vi "DataArray_Formatter.vi"(0 "PartitionArray":string[](array[string]), 1 "Temps":dbl[][](graph), 2 "FrozenFraction":dbl[](array[numeric]), 3 "FreezeTemps":dbl[](array[numeric]), 4 "Offsets":dbl[](array[numeric]), 5 "Offset Applied?":bool, 6 "input cluster":T1={"Core"={"Current VI Reference"=refnum, "Close Panel on Exit?"=FALSE}, "Image Out"=refnum, "State"=0, "Points"={"Top Left"={"X"=0.0, "Y"=0.0}, "Top Right"={"X"=0.0, "Y"=0.0}, "Bottom Left"={"X"=0.0, "Y"=0.0}, "Bottom Right"={"X"=0.0, "Y"=0.0}, "x space 2"=0.0, "y space 2"=0.0, "x_space"=0.0, "y_space"=0.0, "Pixels"=[], "Fixpoint"={"X"=0.0, "Y"=0.0}}, "img_array"=[], "Temps"=[], "Temps_Array"=[], "Scan Area"=0.0, "Fixpoint Area"=0.0, "Config"={"Freezing"={"Cutoff"=2.0, "EndIndex"=2}}, "PCR Size"=0, "ImageCount"=0, "ShowGradient"=FALSE} {"Points"."Bottom Right"."Y" format="%.2f"; "Points"."Bottom Right"."X" format="%.2f"; "Points"."Top Left"."Y" format="%.2f"; "Points"."Top Left"."X" format="%.2f"; "Points"."Top Right"."Y" format="%.2f"; "Points"."Top Right"."X" format="%.2f"; "Points"."Bottom Left"."Y" format="%.2f"; "Points"."Bottom Left"."X" format="%.2f"; "Points"."Fixpoint"."Y" format="%.2f"; "Points"."Fixpoint"."X" format="%.2f"}, 9 "MeltTemps":dbl[](array[numeric])) -> (14 "Data Array":string[][](array[string]))   [LabVIEW 2022 SP3]
uses:
  DataCluster_TCAL.ctl
  <vilib>/vision/Image Controls.llb/IMAQ Image.ctl
  TCE_Config.ctl
panel:
  out "appended array":string[][](array[string])
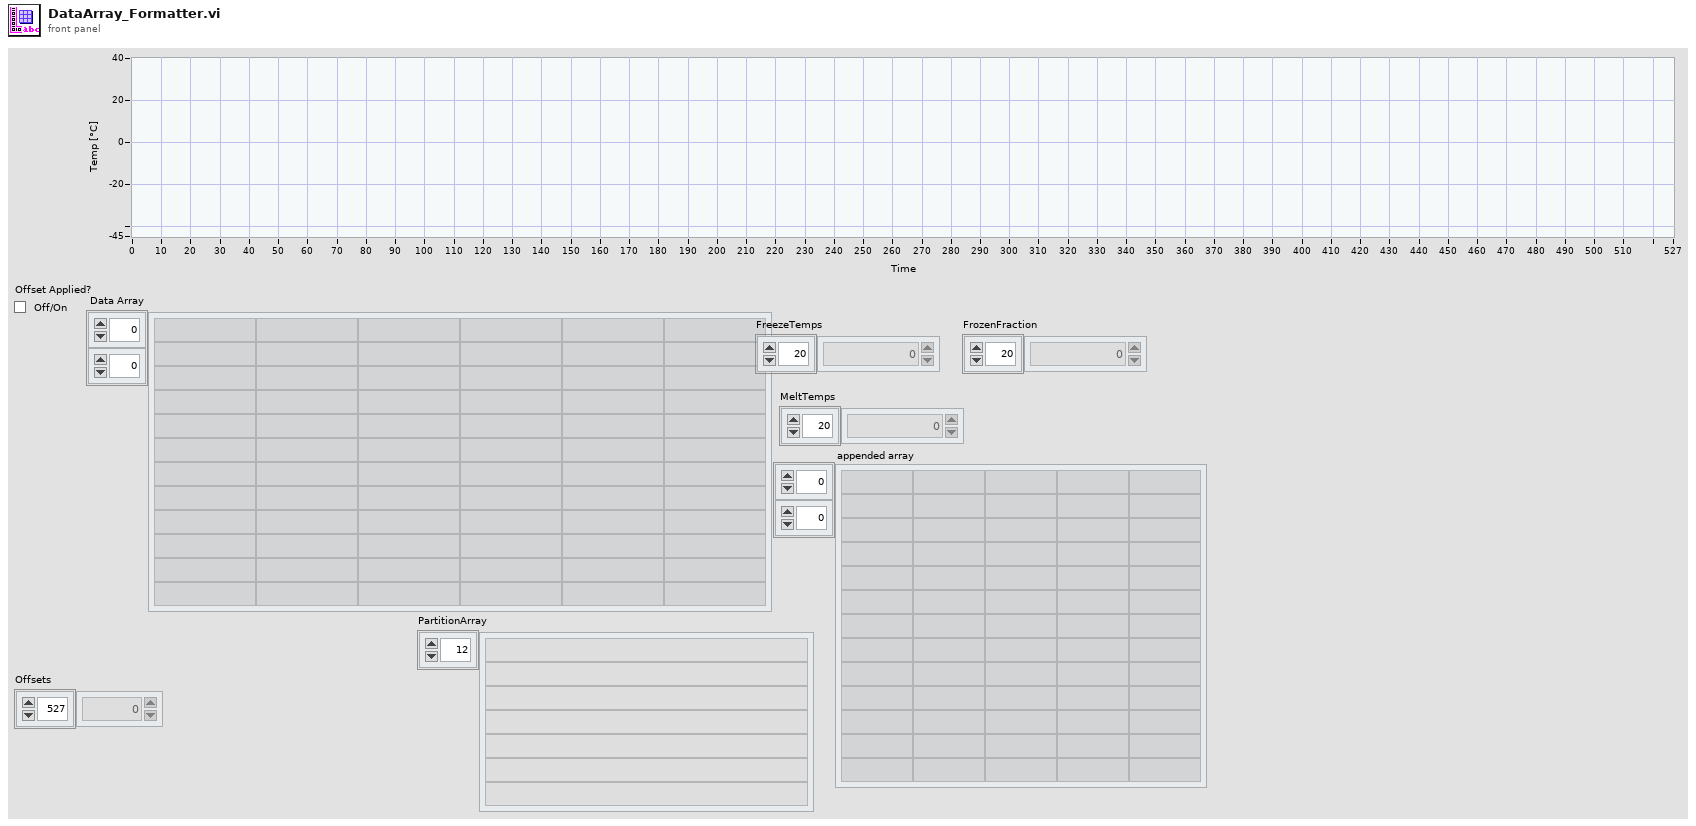
[diagram p1: front panel]
types:
  T1 = typedef "DataCluster_TCAL.ctl" = cluster{"Core":cluster{"Current VI Reference":refnum<vi>, "Close Panel on Exit?":bool}, "Image Out":T2, "State":i32, "Points":cluster{"Top Left":T3, "Top Right":T3, "Bottom Left":T3, "Bottom Right":T3, "x space 2":dbl, "y space 2":sgl, "x_space":sgl, "y_space":sgl, "Pixels":cluster{"X":i32, "Y":i32}[][], "Fixpoint":T3}, "img_array":T2[], "Temps":dbl[], "Temps_Array":dbl[][], "Scan Area":dbl, "Fixpoint Area":dbl, "Config":T4, "PCR Size":u16, "ImageCount":i32, "ShowGradient":bool}
  T2 = typedef "IMAQ Image.ctl" = refnum<image>
  T3 = typedef "IMAQ Point" = cluster{"X":sgl, "Y":sgl}
  T4 = typedef "TCE_Config.ctl" = cluster{"Freezing":cluster{"Cutoff":dbl, "EndIndex":i32}}
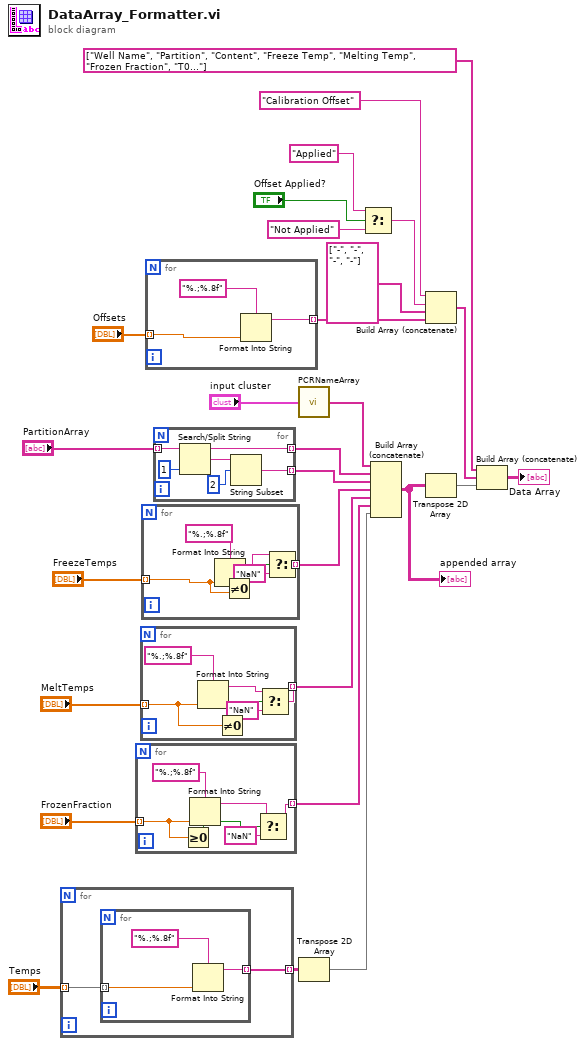
[diagram p0: block diagram]
diagram:
  n1 = for {
    tunnel: "Temps" -> [w29] mode=indexing
    tunnel: [w28] -> w21 mode=indexing
    n2 = for {
      tunnel: w29 -> [w32] mode=indexing
      tunnel: [w31] -> w28 mode=indexing
      n3 = Format Into String(format string="%.;%.8f", w32) -> (resulting string=w31:string)  [unwired: 2 in, 1 out]
    }
  }
  n4 = for {
    tunnel: "FrozenFraction" -> [w35] mode=indexing
    tunnel: [w36] -> w5 mode=indexing
    n5 = Greater Or Equal To 0?(x=w35) -> (x >= 0?=w34:bool)
    n6 = Format Into String(format string="%.;%.8f", w35) -> (resulting string=w37:string)  [unwired: 2 in, 1 out]
    n7 = Select(t=w37, s=w34, f="NaN") -> (s? t:f=w36:string)
  }
  n8 = for {
    tunnel: "MeltTemps" -> [w39] mode=indexing
    tunnel: [w42] -> w10 mode=indexing
    n9 = Format Into String(format string="%.;%.8f", w39) -> (resulting string=w41:string)  [unwired: 2 in, 1 out]
    n10 = Not Equal To 0?(x=w39) -> (x != 0?=w40:bool)
    n11 = Select(t=w41, s=w40, f="NaN") -> (s? t:f=w42:string)
  }
  n12 = for {
    tunnel: "FreezeTemps" -> [w46] mode=indexing
    tunnel: [w49] -> w3 mode=indexing
    n13 = Format Into String(format string="%.;%.8f", w46) -> (resulting string=w48:string)  [unwired: 2 in, 1 out]
    n14 = Not Equal To 0?(x=w46) -> (x != 0?=w47:bool)
    n15 = Select(t=w48, s=w47, f="NaN") -> (s? t:f=w49:string)
  }
  n16 = for {
    tunnel: "Offsets" -> [w53] mode=indexing
    tunnel: [w52] -> w9 mode=indexing
    n17 = Format Into String(format string="%.;%.8f", w53) -> (resulting string=w52:string)  [unwired: 2 in, 1 out]
  }
  n18 = for {
    tunnel: "PartitionArray" -> [w59] mode=indexing
    tunnel: [w55] -> w2 mode=indexing
    tunnel: [w57] -> w1 mode=indexing
    n19 = Search/Split String(string=w59, offset (0)=1) -> (substring before match=w57:string, match + rest of string=w56:string)  [unwired: 1 in, 1 out]
    n20 = String Subset(string=w56, offset (0)=2) -> (substring=w55:string)  [unwired: 1 in]
  }
  n21 = call "PCRNameArray.vi"("input cluster"="input cluster") -> ("WellArray"=w27:string[])
  n22 = Transpose 2D Array(2D array=w21) -> (transposed array=w6:string[][])
  n23 = Select(t="Applied", s="Offset Applied?", f="Not Applied") -> (s? t:f=w12:string)
  n24 = Build Array (concatenate)(w27, w1, w2, w3, w10, w5, w6) -> (w24:string[][])
  "appended array" <- w24
  n25 = Build Array (concatenate)("Calibration Offset" ("element"), w12, string[] ["-", "-", "-", "-"] ("array"), w9) -> (w17:string[])
  n26 = Transpose 2D Array(2D array=w24) -> (transposed array=w23:string[][])
  n27 = Build Array (concatenate)(string[] ["Well Name", "Partition", "Content", "Freeze Temp", "Melting Temp", "Frozen Fraction", "T0..."], w17, w23) -> (→"Data Array":string[][])
